vi "SW_Get_CPU_load_monitor_reference.vi"(2 "error in (no error)":errorcluster) -> (0 "error out":errorcluster, 1 "CPU monitor .NET reference":refnum<k24>)   [LabVIEW 2018, in "Common_Resources.lvlib"]
uses:
  Common_Resources.lvlib
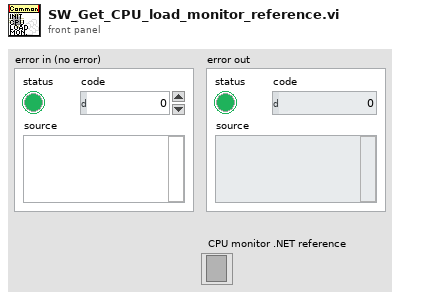
[diagram p1: front panel]
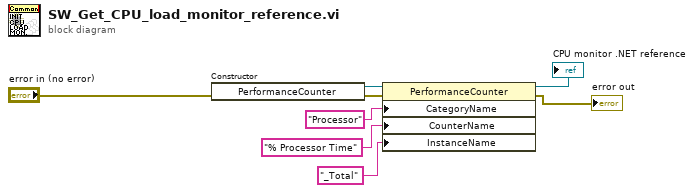
[diagram p0: block diagram]
diagram:
  n1 = constructor class="PerformanceCounter"(error in="error in (no error)") -> (reference out=w3:refnum<k24>, error out=w4:errorcluster)  [unwired: 2 in, 1 out]
  n2 = property class="PerformanceCounter"(reference=w3, error in=w4, "CategoryName"="Processor", "CounterName"="% Processor Time", "InstanceName"="_Total") -> (reference out=→"CPU monitor .NET reference":refnum<k24>, error out=→"error out":errorcluster)
